vi "Demo.vi"() -> ()   [LabVIEW 2020]
uses:
  Worder.lvclass
  config.ctl
  letter_box.ctl
  letter_box_small.ctl
  keyboard.ctl
panel:
  out "number of words":string
  out "keyboard":T1={"A"={"color"=3815996, "char"="A"}, "B"={"color"=3815996, "char"="B"}, "C"={"color"=3815996, "char"="C"}, "D"={"color"=3815996, "char"="D"}, "E"={"color"=3815996, "char"="E"}, "F"={"color"=3815996, "char"="F"}, "G"={"color"=3815996, "char"="G"}, "H"={"color"=3815996, "char"="H"}, "I"={"color"=3815996, "char"="I"}, "J"={"color"=3815996, "char"="J"}, "K"={"color"=3815996, "char"="K"}, "L"={"color"=3815996, "char"="L"}, "M"={"color"=3815996, "char"="M"}, "N"={"color"=3815996, "char"="N"}, "O"={"color"=3815996, "char"="O"}, "P"={"color"=3815996, "char"="P"}, "Q"={"color"=3815996, "char"="Q"}, "R"={"color"=3815996, "char"="R"}, "S"={"color"=3815996, "char"="S"}, "T"={"color"=3815996, "char"="T"}, "U"={"color"=3815996, "char"="U"}, "V"={"color"=3815996, "char"="V"}, "W"={"color"=3815996, "char"="W"}, "X"={"color"=3815996, "char"="X"}, "Y"={"color"=3815996, "char"="Y"}, "Z"={"color"=3815996, "char"="Z"}}
  out "Numeric":i32
  out "gameboard":T3[][](array[typedef])=[[{"color"=16777222, "char"=""}, {"color"=16777222, "char"=""}, {"color"=16777222, "char"=""}, {"color"=16777222, "char"=""}, {"color"=16777222, "char"=""}], [{"color"=16777222, "char"=""}, {"color"=16777222, "char"=""}, {"color"=16777222, "char"=""}, {"color"=16777222, "char"=""}, {"color"=16777222, "char"=""}], [{"color"=16777222, "char"=""}, {"color"=16777222, "char"=""}, {"color"=16777222, "char"=""}, {"color"=16777222, "char"=""}, {"color"=16777222, "char"=""}], [{"color"=16777222, "char"=""}, {"color"=16777222, "char"=""}, {"color"=16777222, "char"=""}, {"color"=16777222, "char"=""}, {"color"=16777222, "char"=""}], [{"color"=16777222, "char"=""}, {"color"=16777222, "char"=""}, {"color"=16777222, "char"=""}, {"color"=16777222, "char"=""}, {"color"=16777222, "char"=""}], [{"color"=16777222, "char"=""}, {"color"=16777222, "char"=""}, {"color"=16777222, "char"=""}, {"color"=16777222, "char"=""}, {"color"=16777222, "char"=""}]]
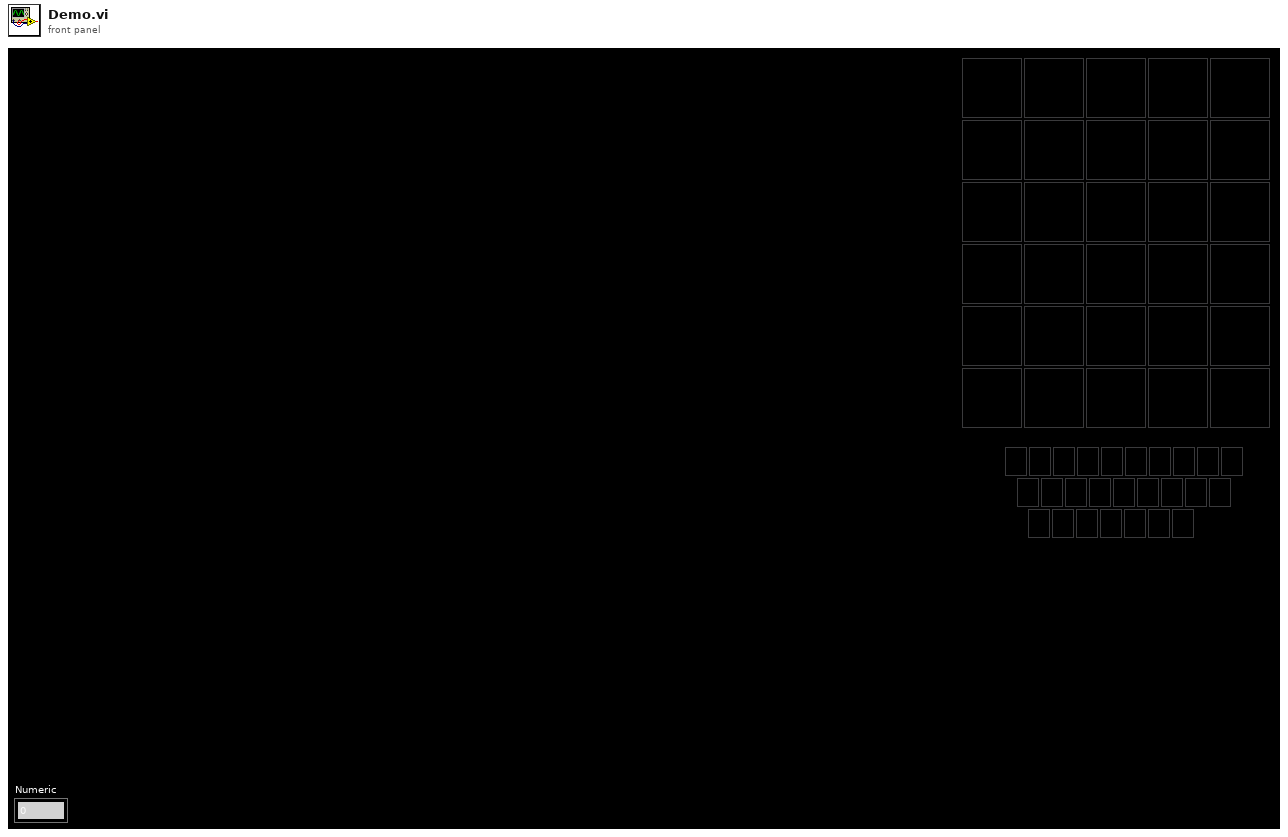
[diagram p1: front panel]
types:
  T1 = typedef "Worder.lvclass/keyboard.ctl" = cluster{"A":T2, "B":T2, "C":T2, "D":T2, "E":T2, "F":T2, "G":T2, "H":T2, "I":T2, "J":T2, "K":T2, "L":T2, "M":T2, "N":T2, "O":T2, "P":T2, "Q":T2, "R":T2, "S":T2, "T":T2, "U":T2, "V":T2, "W":T2, "X":T2, "Y":T2, "Z":T2}
  T2 = typedef "Worder.lvclass/letter_box_small.ctl" = cluster{"color":u32, "char":string}
  T3 = typedef "Worder.lvclass/letter_box.ctl" = cluster{"color":u32, "char":string}
  T4 = typedef "Worder.lvclass/config.ctl" = cluster{"num letters":i32, "num guesses":i32, "default color":u32, "match color":u32, "half match color":u32, "no match color":u32, "dictonary":string[]}
  T5 = typedef "eventvkey.ctl" = enum16{"ASCII", "Enter", "Return", "Shift", "Ctrl", "Alt", "Cmd", "Opt", "Caps", "NumLock", "Clear", "Break", "Up", "Down", "Left", "Right", "Insert", "Delete", "Home", "End", "PageUp", "PageDown", "Escape", "Help", "Pause", "ScrollLock", "F1", "F2", "F3", "F4", "F5", "F6", "F7", "F8", "F9", "F10", "F11", "F12", "F13", "F14", "F15", "F16", "F17", "F18", "F19", "F20", "F21", "F22", "F23", "F24", "Play", "VolumeUp", "VolumeDown", "Mute", "Two Byte Char"}
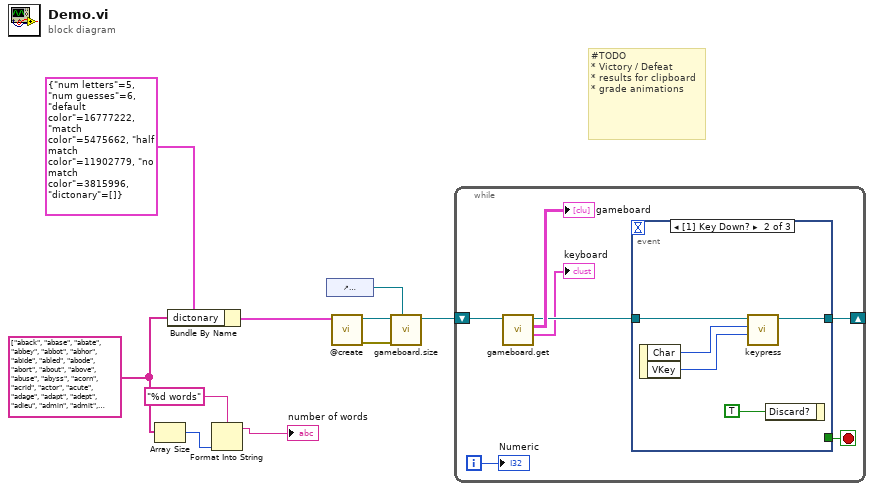
[diagram p0: block diagram]
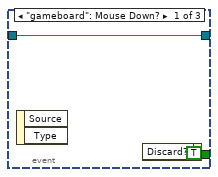
[diagram p2: hidden frame]
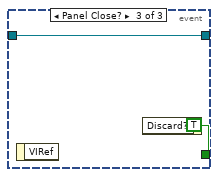
[diagram p3: hidden frame]
diagram:
  w4 = string[] ["aback", "abase", "abate", "abbey", "abbot", "abhor", "abide", "abled", "abode", "abort", "about", "above", "abuse", "abyss", "acorn", "acrid", "actor", "acute", "adage", "adapt", "adept", "adieu", "admin", "admit", "adobe", "adopt", "adore", "adorn", "adult", "affix", "afire", "afoot", "afoul", "after", "again", "agape", "agate", "agent", "agile", "aging", "aglow", "agony", "agora", "agree", "ahead", "aider", "aisle", "alarm", "album", "alert", "algae", "alibi", "alien", "align", "alike", "alive", "allay", "alley", "allot", "allow", "alloy", "aloft", "alone", "along", "aloof", "aloud", "alpha", "altar", "alter", "amass", "amaze", "amber", "amble", "amend", "amiss", "amity", "among", "ample", "amply", "amuse", "angel", "anger", "angle", "angry", "angst", "anime", "ankle", "annex", "annoy", "annul", "anode", "antic", "anvil", "aorta", "apart", "aphid", "aping", "apnea", "apple", "apply", "apron", "aptly", "arbor", "ardor", "arena", "argue", "arise", "armor", "aroma", "arose", "array", "arrow", "arson", "artsy", "ascot", "ashen", "aside", "askew", "assay", "asset", "atoll", "atone", "attic", "audio", "audit", "augur", "aunty", "avail", "avert", "avian", "avoid", "await", "awake", "award", "aware", "awash", "awful", "awoke", "axial", "axiom", "axion", "azure", "bacon", "badge", "badly", "bagel", "baggy", "baker", "baler", "balmy", "banal", "banjo", "barge", "baron", "basal", "basic", "basil", "basin", "basis", "baste", "batch", "bathe", "baton", "batty", "bawdy", "bayou", "beach", "beady", "beard", "beast", "beaut", "beech", "beefy", "befit", "began", "begat", "beget", "begin", "begun", "being", "belch", "belie", "belle", "belly", "below", "bench", "beret", "berry", "berth", "beset", "betel", "bevel", "bezel", "bible", "bicep", "biddy", "bigot", "bilge", "billy", "binge", "bingo", "biome", "birch", "birth", "bison", "bitty", "black", "blade", "blame", "bland", "blank", "blare", "blast", "blaze", "bleak", "bleat", "bleed", "bleep", "blend", "bless", "blimp", "blind", "blink", "bliss", "blitz", "bloat", "block", "bloke", "blond", "blood", "bloom", "blown", "bluer", "bluff", "blunt", "blurb", "blurt", "blush", "board", "boast", "bobby", "boney", "bongo", "bonus", "booby", "boost", "booth", "booty", "booze", "boozy", "borax", "bored", "borne", "bosom", "bossy", "botch", "bough", "boule", "bound", "bowel", "boxer", "brace", "braid", "brain", "brake", "brand", "brash", "brass", "brave", "bravo", "brawl", "brawn", "bread", "break", "breed", "briar", "bribe", "brick", "bride", "brief", "brine", "bring", "brink", "briny", "brisk", "broad", "broil", "broke", "brood", "brook", "broom", "broth", "brown", "brunt", "brush", "brute", "buddy", "budge", "buggy", "bugle", "build", "built", "bulge", "bulky", "bully", "bumpy", "bunch", "bunny", "burly", "burnt", "burst", "bused", "bushy", "butch", "butte", "buxom", "buyer", "bylaw", "cabal", "cabby", "cabin", "cable", "cacao", "cache", "cacti", "caddy", "cadet", "cagey", "cairn", "camel", "cameo", "canal", "candy", "canny", "canoe", "canon", "caper", "caput", "carat", "cargo", "carol", "carry", "carve", "caste", "catch", "cater", "catty", "caulk", "cause", "cavil", "cease", "cedar", "cello", "chafe", "chaff", "chain", "chair", "chalk", "champ", "chant", "chaos", "chard", "charm", "chart", "chase", "chasm", "cheap", "cheat", "check", "cheek", "cheer", "chess", "chest", "chick", "chide", "chief", "child", "chili", "chill", "chime", "china", "chirp", "chock", "choir", "choke", "chord", "chore", "chose", "chuck", "chump", "chunk", "churn", "chute", "cider", "cigar", "cinch", "circa", "civic", "civil", "clack", "claim", "clamp", "clang", "clank", "clash", "clasp", "class", "clean", "clear", "cleat", "cleft", "clerk", "click", "cliff", "climb", "cling", "clink", "cloak", "clock", "clone", "close", "cloth", "cloud", "clout", "clove", "clown", "cluck", "clued", "clump", "clung", "coach", "coast", "cobra", "cocoa", "colon", "color", "comet", "comfy", "comic", "comma", "conch", "condo", "conic", "copse", "coral", "corer", "corny", "couch", "cough", "could", "count", "coupe", "court", "coven", "cover", "covet", "covey", "cower", "coyly", "crack", "craft", "cramp", "crane", "crank", "crash", "crass", "crate", "crave", "crawl", "craze", "crazy", "creak", "cream", "credo", "creed", "creek", "creep", "creme", "crepe", "crept", "cress", "crest", "crick", "cried", "crier", "crime", "crimp", "crisp", "croak", "crock", "crone", "crony", "crook", "cross", "croup", "crowd", "crown", "crude", "cruel", "crumb", "crump", "crush", "crust", "crypt", "cubic", "cumin", "curio", "curly", "curry", "curse", "curve", "curvy", "cutie", "cyber", "cycle", "cynic", "daddy", "daily", "dairy", "daisy", "dally", "dance", "dandy", "datum", "daunt", "dealt", "death", "debar", "debit", "debug", "debut", "decal", "decay", "decor", "decoy", "decry", "defer", "deign", "deity", "delay", "delta", "delve", "demon", "demur", "denim", "dense", "depot", "depth", "derby", "deter", "detox", "deuce", "devil", "diary", "dicey", "digit", "dilly", "dimly", "diner", "dingo", "dingy", "diode", "dirge", "dirty", "disco", "ditch", "ditto", "ditty", "diver", "dizzy", "dodge", "dodgy", "dogma", "doing", "dolly", "donor", "dont", "donut", "dopey", "doubt", "dough", "dowdy", "dowel", "downy", "dowry", "dozen", "draft", "drain", "drake", "drama", "drank", "drape", "drawl", "drawn", "dread", "dream", "dress", "dried", "drier", "drift", "drill", "drink", "drive", "droit", "droll", "drone", "drool", "droop", "dross", "drove", "drown", "druid", "drunk", "dryer", "dryly", "duchy", "dully", "dummy", "dumpy", "dunce", "dusky", "dusty", "dutch", "duvet", "dwarf", "dwell", "dwelt", "dying", "eager", "eagle", "early", "earns", "earth", "easel", "eaten", "eater", "ebony", "eclat", "edict", "edify", "eerie", "egret", "eight", "eject", "eking", "elate", "elbow", "elder", "elect", "elegy", "elfin", "elide", "elite", "elope", "elude", "email", "embed", "ember", "emcee", "empty", "enact", "endow", "enema", "enemy", "enjoy", "ennui", "ensue", "enter", "entry", "envoy", "epoch", "epost", "epoxy", "equal", "equip", "erase", "erect", "erode", "error", "erupt", "essay", "ester", "ether", "ethic", "ethos", "etude", "evade", "event", "every", "evict", "evoke", "exact", "exalt", "excel", "exert", "exile", "exist", "expel", "extol", "extra", "exult", "eying", "fable", "facet", "faint", "fairy", "faith", "false", "fancy", "fanny", "farce", "farts", "fatal", "fatty", "fault", "fauna", "favor", "feast", "fecal", "feign", "fella", "felon", "femme", "femur", "fence", "feral", "ferry", "fetal", "fetch", "fetid", "fetus", "fever", "fewer", "fiber", "fibre", "ficus", "field", "fiend", "fiery", "fifth", "fifty", "fight", "filer", "filet", "filly", "filmy", "filth", "final", "finch", "finer", "first", "fishy", "fixer", "fizzy", "fjord", "flack", "flail", "flair", "flake", "flaky", "flame", "flank", "flare", "flash", "flask", "fleck", "fleet", "flesh", "flick", "flier", "fling", "flint", "flirt", "float", "flock", "flood", "floor", "flora", "floss", "flour", "flout", "flown", "fluff", "fluid", "fluke", "flume", "flung", "flunk", "flush", "flute", "flyer", "foamy", "focal", "focus", "foggy", "foist", "folio", "folly", "foray", "force", "forge", "forgo", "forte", "forth", "forty", "forum", "found", "foyer", "frail", "frame", "frank", "fraud", "freak", "freed", "freer", "fresh", "friar", "fried", "frill", "frisk", "fritz", "frock", "frond", "front", "frost", "froth", "frown", "froze", "fruit", "fudge", "fugue", "fully", "fungi", "funky", "funny", "furor", "furry", "fussy", "fuzzy", "gaffe", "gaily", "gamer", "gamma", "gamut", "gassy", "gaudy", "gauge", "gaunt", "gauze", "gavel", "gawky", "gayer", "gayly", "gazer", "gecko", "geeky", "geese", "genie", "genre", "ghost", "ghoul", "giant", "giddy", "gipsy", "girly", "girth", "given", "giver", "glade", "gland", "glare", "glass", "glaze", "gleam", "glean", "glide", "glint", "gloat", "globe", "gloom", "glory", "gloss", "glove", "glyph", "gnash", "gnome", "godly", "going", "golem", "golly", "gonad", "goner", "goody", "gooey", "goofy", "goose", "gorge", "gouge", "gourd", "grace", "grade", "graft", "grail", "grain", "grand", "grant", "grape", "graph", "grasp", "grass", "grate", "grave", "gravy", "graze", "great", "greed", "green", "greet", "grief", "grill", "grime", "grimy", "grind", "gripe", "groan", "groin", "groom", "grope", "gross", "group", "grout", "grove", "growl", "grown", "gruel", "gruff", "grunt", "guard", "guava", "guess", "guest", "guide", "guild", "guile", "guilt", "guise", "gulch", "gully", "gumbo", "gummy", "guppy", "gusto", "gusty", "gypsy", "habit", "hairy", "halve", "handy", "happy", "hardy", "harem", "harpy", "harry", "harsh", "haste", "hasty", "hatch", "hater", "haunt", "haute", "haven", "havoc", "hazel", "heady", "heard", "heart", "heath", "heave", "heavy", "hedge", "hefty", "heist", "helix", "hello", "hence", "henry", "heron", "hilly", "hinge", "hippo", "hippy", "hitch", "hoard", "hobby", "hoist", "holly", "homer", "honey", "honor", "horde", "horny", "horse", "hotel", "hotly", "hound", "house", "hovel", "hover", "howdy", "human", "humid", "humor", "humph", "humus", "hunch", "hunky", "hurry", "husky", "hussy", "hutch", "hydro", "hyena", "hymen", "hyper", "icily", "icing", "ideal", "ideas", "idiom", "idiot", "idler", "idyll", "igloo", "iliac", "image", "imbue", "impel", "imply", "inane", "inbox", "incur", "index", "inept", "inert", "infer", "ingot", "inlay", "inlet", "inner", "input", "inter", "intro", "ionic", "irate", "irony", "islet", "issue", "itchy", "ivory", "japan", "jaunt", "jazzy", "jelly", "jerky", "jetty", "jewel", "jiffy", "joint", "joist", "joker", "jolly", "jones", "joust", "judge", "juice", "juicy", "jumbo", "jumpy", "junta", "junto", "juror", "kappa", "karma", "kayak", "kebab", "khaki", "kinky", "kiosk", "kitty", "knack", "knave", "knead", "kneed", "kneel", "knelt", "knife", "knock", "knoll", "known", "koala", "krill", "label", "labor", "laden", "ladle", "lager", "lance", "lanky", "lapel", "lapse", "large", "larva", "lasso", "latch", "later", "lathe", "latte", "laugh", "laura", "layer", "leach", "leafy", "leaky", "leant", "leapt", "learn", "lease", "leash", "least", "leave", "ledge", "leech", "leery", "lefty", "legal", "leggy", "lemon", "lemur", "leper", "level", "lever", "lewis", "libel", "liege", "light", "liken", "lilac", "limbo", "limit", "linen", "liner", "lingo", "lipid", "lithe", "liver", "livid", "llama", "loamy", "loath", "lobby", "local", "locus", "lodge", "lofty", "logic", "login", "loopy", "loose", "lorry", "loser", "louse", "lousy", "lover", "lower", "lowly", "loyal", "lucid", "lucky", "lumen", "lumpy", "lunar", "lunch", "lunge", "lupus", "lurch", "lurid", "lusty", "lying", "lymph", "lynch", "lyric", "macaw", "macho", "macro", "madam", "madly", "mafia", "magic", "magma", "maize", "major", "maker", "mambo", "mamma", "mammy", "manga", "mange", "mango", "mangy", "mania", "manic", "manly", "manor", "maple", "march", "marry", "marsh", "mason", "masse", "match", "matey", "mauve", "maxim", "maybe", "mayor", "mealy", "meant", "meany", "meats", "meaty", "mecca", "medal", "media", "medic", "melee", "melon", "mercy", "merge", "merit", "merry", "metal", "meter", "metro", "micro", "midge", "midst", "might", "milky", "mimic", "mince", "miner", "minim", "minor", "minty", "minus", "mirth", "miser", "missy", "mocha", "modal", "model", "modem", "mogul", "moist", "molar", "moldy", "money", "month", "moody", "moose", "moral", "moron", "morph", "mossy", "motel", "motif", "motor", "motto", "moult", "mound", "mount", "mourn", "mouse", "mousy", "mouth", "mover", "movie", "mower", "mucky", "mucus", "muddy", "mulch", "mummy", "munch", "mural", "murky", "mushy", "music", "musky", "musty", "myrrh", "nadir", "nails", "naive", "nanny", "nasal", "nasty", "natal", "naval", "navel", "needy", "neigh", "nerdy", "nerve", "never", "newer", "newly", "nicer", "niche", "niece", "night", "ninja", "ninny", "ninth", "noble", "nobly", "noise", "noisy", "nomad", "noose", "north", "nosey", "notch", "notes", "novel", "nudge", "nurse", "nutty", "nylon", "nymph", "oaken", "obese", "occur", "ocean", "octal", "octet", "odder", "oddly", "offal", "offer", "often", "olden", "older", "olive", "ombre", "omega", "onery", "onion", "onset", "opera", "opine", "opium", "optic", "orbit", "order", "organ", "other", "otter", "ought", "ounce", "outdo", "outer", "outgo", "ovary", "ovate", "overt", "ovine", "ovoid", "owing", "owner", "oxide", "ozone", "paddy", "pagan", "paint", "paler", "palsy", "panel", "panic", "pansy", "papal", "paper", "parer", "parka", "parry", "parse", "party", "pasta", "paste", "pasty", "patch", "patio", "patsy", "patty", "pause", "payee", "payer", "peace", "peach", "pearl", "pears", "pecan", "pedal", "penal", "pence", "penne", "penny", "perch", "peril", "perky", "pesky", "pesto", "petal", "peter", "petty", "phase", "phone", "phony", "photo", "piano", "picky", "piece", "piety", "piggy", "pilot", "pinch", "piney", "pinky", "pinto", "piper", "pique", "pitch", "pithy", "pivot", "pixel", "pixie", "pizza", "place", "plaid", "plain", "plait", "plane", "plank", "plant", "plate", "plaza", "plead", "pleat", "plied", "plier", "pluck", "plumb", "plume", "plump", "plunk", "plush", "poesy", "point", "poise", "poker", "polar", "polka", "polyp", "pooch", "poppy", "porch", "ports", "poser", "posit", "posse", "pouch", "pound", "pouty", "power", "prank", "prawn", "preen", "press", "price", "prick", "pride", "pried", "prime", "primo", "print", "prior", "prism", "privy", "prize", "probe", "prone", "prong", "proof", "prose", "proud", "prove", "prowl", "proxy", "prude", "prune", "psalm", "pubic", "pudgy", "puffy", "pulpy", "pulse", "punch", "pupal", "pupil", "puppy", "puree", "purer", "purge", "purse", "pushy", "putty", "pygmy", "quack", "quail", "quake", "qualm", "quark", "quart", "quash", "quasi", "queen", "queer", "quell", "query", "quest", "queue", "quick", "quiet", "quill", "quilt", "quirk", "quite", "quota", "quote", "quoth", "qwoop", "rabbi", "rabid", "racer", "radar", "radii", "radio", "rages", "rains", "rainy", "raise", "rajah", "rally", "ralph", "ramen", "ranch", "randy", "range", "rapid", "rarer", "raspy", "rates", "ratio", "ratty", "raven", "rayon", "razor", "reach", "react", "ready", "realm", "rearm", "rebar", "rebel", "rebus", "rebut", "recap", "recur", "recut", "reedy", "refer", "refit", "regal", "rehab", "reign", "relax", "relay", "relic", "remit", "renal", "renew", "rents", "repay", "repel", "reply", "rerun", "reset", "resin", "retch", "retro", "retry", "reuse", "revel", "revue", "rhino", "rhyme", "rider", "ridge", "rifle", "right", "rigid", "rigor", "rinse", "ripen", "riper", "risen", "riser", "risky", "rival", "river", "rivet", "roach", "roast", "robin", "robot", "rocky", "rodeo", "roger", "rogue", "roomy", "roost", "rotor", "rouge", "rough", "round", "rouse", "route", "rover", "rowdy", "rower", "royal", "ruddy", "ruder", "rugby", "ruler", "rumba", "rumor", "rumpf", "rupee", "rusty", "sabre", "sadly", "safer", "saint", "salad", "sally", "salon", "salsa", "salty", "salve", "salvo", "sandy", "saner", "sappy", "sassy", "satin", "satyr", "sauce", "saucy", "sauna", "saute", "savor", "savoy", "savvy", "scald", "scale", "scalp", "scaly", "scamp", "scant", "scare", "scarf", "scary", "scene", "scent", "scion", "scoff", "scold", "scone", "scoop", "scope", "score", "scorn", "scour", "scout", "scowl", "scram", "scrap", "scree", "screw", "scrub", "scrum", "scuba", "sedan", "seedy", "segue", "seize", "semen", "sense", "sepia", "serif", "serum", "serve", "setup", "seven", "sever", "sewer", "shack", "shade", "shady", "shaft", "shake", "shaky", "shale", "shall", "shalt", "shame", "shank", "shape", "shard", "share", "shark", "sharp", "shawl", "shear", "sheen", "sheep", "sheer", "sheet", "sheik", "shelf", "shell", "shied", "shift", "shine", "shiny", "shire", "shirk", "shirt", "shoal", "shock", "shone", "shook", "shoot", "shore", "shorn", "short", "shout", "shove", "shown", "showy", "shrew", "shrub", "shrug", "shuck", "shunt", "shush", "shyly", "siege", "sieve", "sight", "sigma", "silky", "silly", "simon", "since", "sinew", "singe", "siren", "sissy", "sixth", "sixty", "skate", "skier", "skiff", "skill", "skimp", "skirt", "skulk", "skull", "skunk", "slack", "slain", "slang", "slant", "slash", "slate", "slave", "sleek", "sleep", "sleet", "slept", "slice", "slick", "slide", "slime", "slimy", "sling", "slink", "sloop", "slope", "slosh", "sloth", "slump", "slung", "slunk", "slurp", "slush", "slyly", "smack", "small", "smart", "smash", "smear", "smell", "smelt", "smile", "smirk", "smite", "smith", "smock", "smoke", "smoky", "smote", "snack", "snail", "snake", "snaky", "snare", "snarl", "sneak", "sneer", "snide", "sniff", "snipe", "snoop", "snore", "snort", "snout", "snowy", "snuck", "snuff", "soapy", "soare", "sober", "soggy", "solar", "solid", "solve", "sonar", "sonic", "sooth", "sooty", "sorry", "sound", "south", "sower", "space", "spade", "spank", "spare", "spark", "spasm", "spawn", "speak", "spear", "speck", "speed", "spell", "spelt", "spend", "spent", "sperm", "spice", "spicy", "spied", "spiel", "spike", "spiky", "spill", "spilt", "spine", "spiny", "spire", "spite", "splat", "split", "spoil", "spoke", "spoof", "spook", "spool", "spoon", "spore", "sport", "spout", "spray", "spree", "sprig", "spunk", "spurn", "spurt", "squad", "squat", "squib", "stack", "staff", "stage", "staid", "stain", "stair", "stake", "stale", "stalk", "stall", "stamp", "stand", "stank", "stare", "stark", "start", "stash", "state", "stave", "stead", "steak", "steal", "steam", "steed", "steel", "steep", "steer", "stein", "stern", "stick", "stiff", "still", "stilt", "sting", "stink", "stint", "stock", "stoic", "stoke", "stole", "stomp", "stone", "stony", "stood", "stool", "stoop", "store", "stork", "storm", "story", "stout", "stove", "strap", "straw", "stray", "strip", "strut", "stuck", "study", "stuff", "stump", "stung", "stunk", "stunt", "style", "suave", "sugar", "suing", "suite", "sulky", "sully", "sumac", "sunny", "super", "surer", "surge", "surly", "sushi", "swami", "swamp", "swarm", "swash", "swath", "swear", "sweat", "sweep", "sweet", "swell", "swept", "swift", "swill", "swine", "swing", "swirl", "swish", "swoon", "swoop", "sword", "swore", "sworn", "swung", "synod", "syrup", "tabby", "table", "taboo", "tacit", "tacky", "taffy", "taint", "taken", "taker", "tales", "tally", "talon", "tamer", "tango", "tangy", "taper", "tapir", "tardy", "tarot", "taste", "tasty", "tatty", "taunt", "tawny", "teach", "teams", "tears", "teary", "tease", "teddy", "teeth", "tempo", "tenet", "tenor", "tense", "tenth", "tepee", "tepid", "terra", "terry", "terse", "testy", "thank", "theft", "their", "theme", "there", "these", "theta", "thick", "thief", "thigh", "thing", "think", "third", "thong", "thorn", "those", "three", "threw", "throb", "throw", "thrum", "thumb", "thump", "thyme", "tiara", "tibia", "tidal", "tiger", "tight", "tilde", "timer", "timid", "tipsy", "tired", "titan", "tithe", "title", "toast", "today", "toddy", "token", "tonal", "tonga", "tonic", "tooth", "topaz", "topic", "torch", "torso", "torus", "total", "totem", "touch", "tough", "towel", "tower", "toxic", "toxin", "trace", "track", "tract", "trade", "trail", "train", "trait", "tramp", "trash", "trawl", "tread", "treat", "trend", "triad", "trial", "tribe", "trice", "trick", "tried", "tripe", "trite", "troll", "troop", "trope", "trout", "trove", "truce", "truck", "truer", "truly", "trunk", "truss", "trust", "truth", "tryst", "tubal", "tuber", "tulip", "tulle", "tumor", "tunic", "turbo", "tutor", "twang", "tweak", "tweed", "tweet", "twice", "twine", "twirl", "twist", "twixt", "tying", "udder", "ulcer", "ultra", "umbra", "uncle", "uncut", "under", "undid", "undue", "unfed", "unfit", "unify", "union", "unite", "unity", "unlit", "unmet", "unset", "untie", "until", "unwed", "unzip", "upper", "upset", "urban", "urine", "usage", "usher", "using", "usual", "usurp", "utile", "utter", "vague", "valet", "valid", "valor", "value", "valve", "vapid", "vapor", "vault", "vaunt", "vegan", "venom", "venue", "verge", "verse", "verso", "verve", "vicar", "video", "vigil", "vigor", "villa", "vinyl", "viola", "viper", "viral", "virus", "visit", "visor", "vista", "vital", "vivid", "vixen", "vocal", "vodka", "vogue", "voice", "voila", "vomit", "voter", "vouch", "vowel", "vying", "wacky", "wafer", "wager", "wagon", "waist", "waive", "waltz", "warty", "waste", "watch", "water", "waver", "waxen", "weary", "weave", "wedge", "weedy", "weigh", "weird", "welch", "welsh", "wench", "whack", "whale", "wharf", "wheat", "wheel", "whelp", "where", "which", "whiff", "while", "whine", "whiny", "whirl", "whisk", "white", "whole", "whoop", "whose", "widen", "wider", "widow", "width", "wield", "wight", "willy", "wimpy", "wince", "winch", "windy", "wiser", "wispy", "witch", "witty", "woken", "woman", "women", "woody", "wooer", "wooly", "woozy", "wordy", "world", "worry", "worse", "worst", "worth", "would", "wound", "woven", "wrack", "wrath", "wreak", "wreck", "wrest", "wring", "wrist", "write", "wrong", "wrote", "wrung", "wryly", "yacht", "yearn", "yeast", "yield", "young", "youth", "zebra", "zesty", "zonal", "shard", "sharp", "choir", "meats", "steam", "prick", "reach", "rates", "slate", "abyss", "steep", "creep", "minor", "rains", "bumpy", "sabre", "qwoop", "other", "nails", "charm", "graph"]
  # "#TODO\n* Victory / Defeat\n* results for clipboard\n* grade animations"
  n1 = Array Size(array=w4) -> (size(s)=w3:i32)
  n2 = Bundle By Name(cluster=T4 {"num letters"=5, "num guesses"=6, "default color"=16777222, "match color"=5475662, "half match color"=11902779, "no match color"=3815996, "dictonary"=[]} ("config"), "dictonary"=w4) -> (w9:T4)
  n3 = Format Into String(format string="%d words", w3) -> (resulting string=→"number of words":string)  [unwired: 2 in, 1 out]
  n4 = control-ref of="gameboard"() -> (w6:refnum<vi>)
  n5 = call "@create.vi"("config"=w9) -> ("error out"=w7:errorcluster, "Worder out"=w8:refnum<class "Worder.lvclass">)  [unwired: 9 in]
  n6 = call "gameboard.size.vi"("gameboard ref"=w6, "error in (no error)"=w7, "Worder in"=w8) -> ("Worder out"=w5:refnum<class "Worder.lvclass">)  [unwired: 7 in, 1 out]
  n7 = while {
    shift-right: [w12] -> _
    shift-left: w5 -> [w14]
    i -> [w16]
    stop <- w17 stop-if-true
    n8 = call "gameboard.get.vi"("Worder in"=w14) -> ("keyboard"=→"keyboard":T1, "gameboard"=→"gameboard":T3[][], "Worder out"=w13:refnum<class "Worder.lvclass">)  [unwired: 8 in]
    n9 = event shown="[1] Key Down?" {
      selector: _ -> [_ _ _]
      dyn-events: _ -> [_ _ _]
      timeout: _ -> [_ _ _]
      tunnel: [_ _ w26] -> w17
      tunnel: w13 -> [w18 w21 w25]
      tunnel: [w18 w22 w25] -> w12
      event "gameboard": Mouse Down? {
        n10 = event-data() -> ()  [unwired: 1 in, 2 out]
        n11 = event-data("Discard?"=TRUE) -> ()  [unwired: 1 in, 1 out]
      }
      event Key Down? {
        n12 = event-data() -> ("Char"=w23:i16, "VKey"=w20:T5)  [unwired: 1 in]
        n13 = call "keypress.vi"("VKey"=w20, "Char"=w23, "Worder in"=w21) -> ("Worder out"=w22:refnum<class "Worder.lvclass">)  [unwired: 7 in, 1 out]
        n14 = event-data("Discard?"=TRUE) -> ()  [unwired: 1 in, 1 out]
      }
      event Panel Close? {
        w26 = TRUE ("Discard?")
        n15 = event-data() -> ()  [unwired: 1 in, 1 out]
        n16 = event-data("Discard?"=w26) -> ()  [unwired: 1 in, 1 out]
      }
    }
    "Numeric" <- w16
  }
